vi "MOSES Background 4.vi"(5 "Array Input":refnum<vi>) -> (0 "PSU":dbl[](graph), 1 "Values to Output":T1, 2 "Power Supply Filter Input":dbl[](graph), 3 "ROE":dbl[](graph))   [LabVIEW 2013]
uses:
  Instance          20 26Saved   MOSES Background 4 .vi
  Instance          18 26Saved   MOSES Background 4 .vi
  Instance           7 26Saved   MOSES Background 4 .vi
  Instance          15 26Saved   MOSES Background 4 .vi
  Instance          22 26Saved   MOSES Background 4 .vi
  Instance          13 26Saved   MOSES Background 4 .vi
  Instance          11 26Saved   MOSES Background 4 .vi
  Instance           9 26Saved   MOSES Background 4 .vi
  Instance           5 26Saved   MOSES Background 4 .vi
  Instance           3 26Saved   MOSES Background 4 .vi
  Instance          26 26Saved   MOSES Background 4 .vi
  Instance          25 26Saved   MOSES Background 4 .vi
  Instance          30 26Saved   MOSES Background 4 .vi
  Instance          28 26Saved   MOSES Background 4 .vi
  <vilib>/express/express arith-compare/Formula/XNode/ExpressFormulaBlockNode.xnode
panel:
  out "Boolean 17":bool
  out "Boolean 16":bool
  out "Boolean 15":bool
  out "Boolean 14":bool
  out "Boolean 13":bool
  out "Boolean 41":bool
  out "Boolean 40":bool
  out "Boolean 39":bool
  out "Boolean 38":bool
  out "Boolean 37":bool
  out "Boolean 36":bool
  out "Boolean 35":bool
  out "Boolean 34":bool
  out "Boolean 33":bool
  out "Boolean 32":bool
  out "Boolean 12":bool
  out "Boolean 11":bool
  out "Boolean 10":bool
  out "Boolean 84":bool
  out "Boolean 83":bool
  out "T_PSU, PSU Temp.":dbl
  out "Boolean 82":bool
  out "Boolean 81":bool
  out "T_ROE, ROE Temp.":dbl
  in  "stop 4":bool
  out "ROE_PSI, ROE power supply input current":dbl
  out "ROE_PSV, ROE power supply input voltage":dbl
  out "I_pf5, Premod filter 5V input current":dbl
  out "HAFI, H-alpha filter current":dbl
  out "S28I, Shutter 28V power current":dbl
  out "Ipf12+, Premod filter positive 12V input current":dbl
  out "If_in":dbl[](graph)
  out "Boolean 31":bool
  out "Boolean 30":bool
  out "Boolean 29":bool
  out "If_in, Power supply filter input current":dbl
  out "Boolean 23":bool
  out "Boolean 22":bool
  out "Boolean 9":bool
  out "Boolean 8":bool
  out "Boolean 7":bool
  out "HACV, H-alpha camera voltage":dbl
  out "HAFV, H-alpha filter voltage":dbl
  out "Boolean 21":bool
  out "Boolean 20":bool
  out "Boolean 19":bool
  out "Boolean 18":bool
  out "S28V, Shutter 28V power voltage":dbl
  out "T5V, Thermal 5V power voltage":dbl
  out "V5s, MGA2805S output voltage":dbl
  out "Vina_0y":dbl
  out "Vina_-y":dbl
  out "Vina_+y, INA330 Output":dbl
  out "Vex_0y":dbl
  out "Vex_-y":dbl
  out "Vex_+y":dbl
  out "Va_0y":dbl
  out "Va_-y":dbl
  out "Waveform Chart 2":dbl[](graph)
  out "Va_+y, Thermistor Voltage":dbl
  # "A"
  # "A"
  # "V"
  # "mA"
  # "C"
  # "C"
  # "V"
  # "V"
  # "V"
  # "V"
  # "V"
  # "A"
  # "mA"
  # "mA"
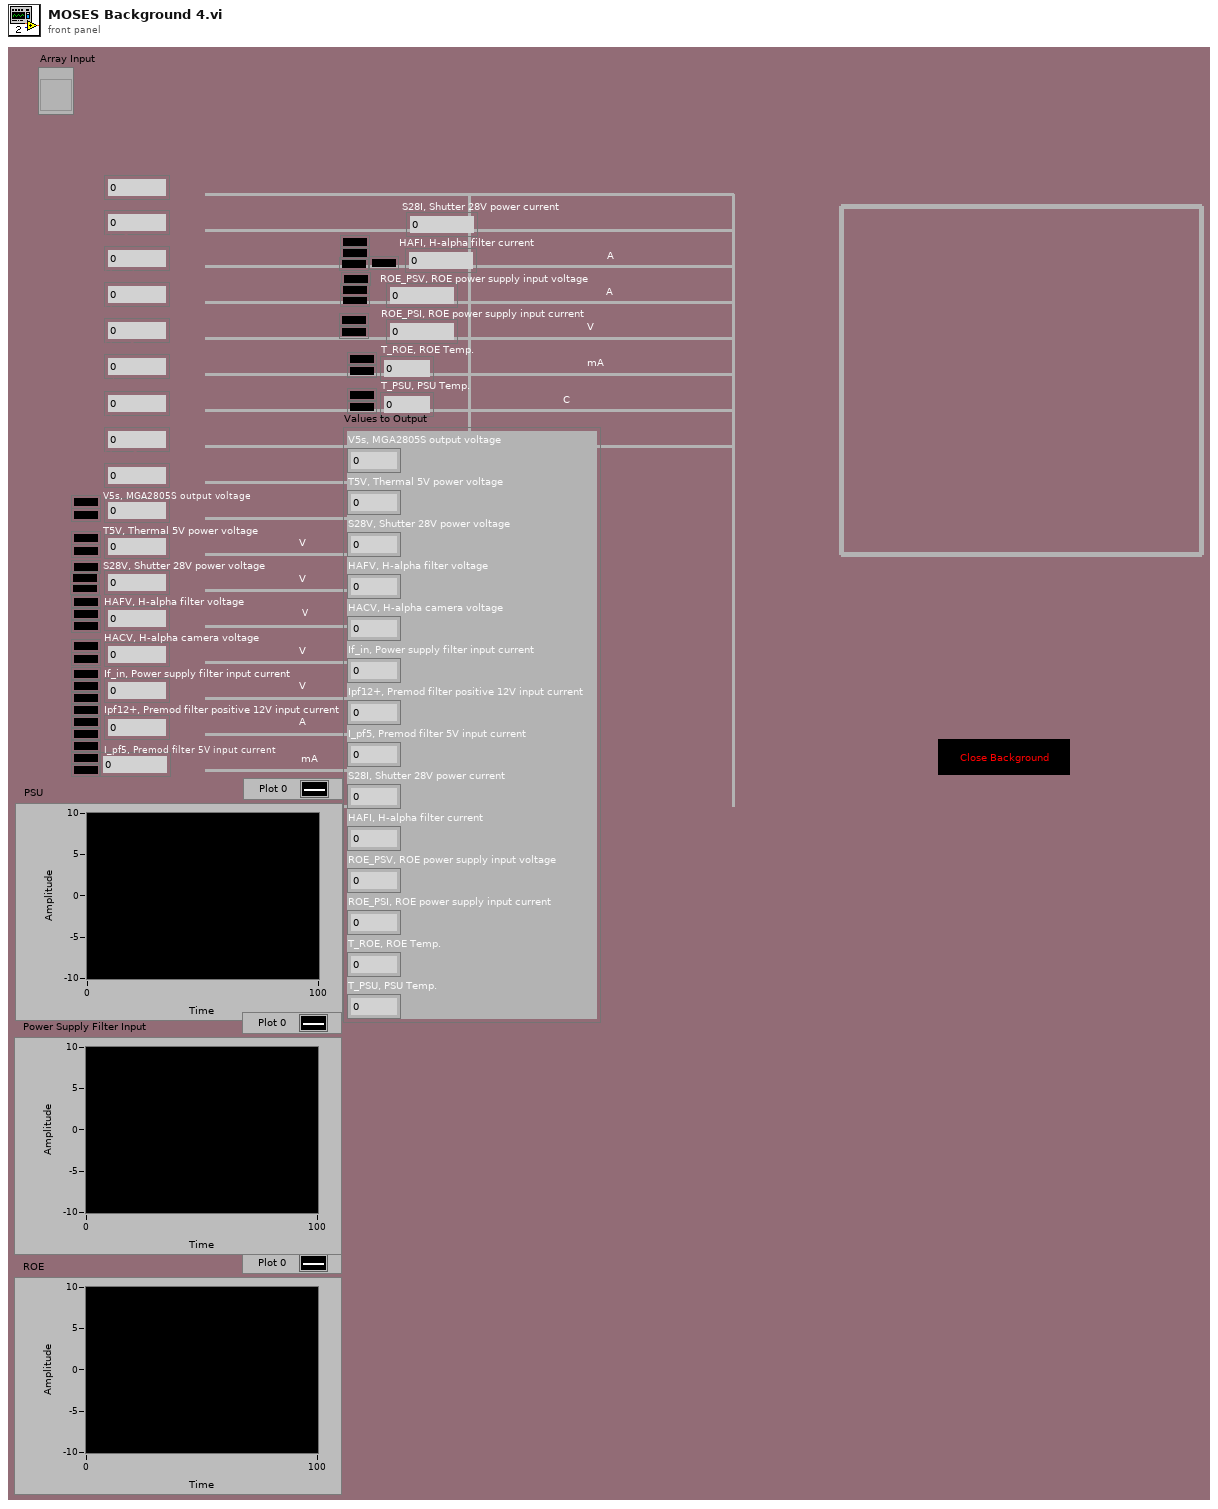
[diagram p1: front panel]
types:
  T1 = cluster{"V5s, MGA2805S output voltage":dbl, "T5V, Thermal 5V power voltage":dbl, "S28V, Shutter 28V power voltage":dbl, "HAFV, H-alpha filter voltage":dbl, "HACV, H-alpha camera voltage":dbl, "If_in, Power supply filter input current":dbl, "Ipf12+, Premod filter positive 12V input current":dbl, "I_pf5, Premod filter 5V input current":dbl, "S28I, Shutter 28V power current":dbl, "HAFI, H-alpha filter current":dbl, "ROE_PSV, ROE power supply input voltage":dbl, "ROE_PSI, ROE power supply input current":dbl, "T_ROE, ROE Temp.":dbl, "T_PSU, PSU Temp.":dbl}
  T2 = cluster{"Value[0]":dbl, "Value[1]":dbl, "Value[2]":dbl, "Value[3]":dbl, "Value[4]":dbl, "Value[5]":dbl, "Value[6]":dbl, "Value[7]":dbl, "Value[8]":dbl, "Value[9]":dbl, "Value[10]":dbl, "Value[11]":dbl, "Value[12]":dbl, "Value[13]":dbl, "Value[14]":dbl, "Value[15]":dbl, "Value[16]":dbl, "Value[17]":dbl, "Value[18]":dbl, "Value[19]":dbl, "Value[20]":dbl, "Value[21]":dbl, "Value[22]":dbl, "Value[23]":dbl, "Value[24]":dbl, "Value[25]":dbl, "Value[26]":dbl, "Value[27]":dbl, "Value[28]":dbl, "Value[29]":dbl, "Value[30]":dbl, "Value[31]":dbl, "Value[32]":dbl, "Value[33]":dbl, "Value[34]":dbl, "Value[35]":dbl, "Value[36]":dbl, "Value[37]":dbl, "Value[38]":dbl, "Value[39]":dbl, "Value[40]":dbl, "Value[41]":dbl, "Value[42]":dbl, "Value[43]":dbl, "Value[44]":dbl, "Value[45]":dbl, "Value[46]":dbl, "Value[47]":dbl, "Value[48]":dbl, "Value[49]":dbl, "Value[50]":dbl, "Value[51]":dbl, "Value[52]":dbl, "Value[53]":dbl, "Value[54]":dbl, "Value[55]":dbl, "Value[56]":dbl, "Value[57]":dbl, "Value[58]":dbl, "Value[59]":dbl, "Value[60]":dbl, "Value[61]":dbl, "Value[62]":dbl, "Value[63]":dbl, "Value[64]":dbl, "Value[65]":dbl, "Value[66]":dbl, "Value[67]":dbl, "Value[68]":dbl, "Value[69]":dbl}
  T3 = cluster{"[0]":dbl, "[1]":dbl, "[2]":dbl, "[3]":dbl, "[4]":dbl, "[5]":dbl, "[6]":dbl, "[7]":dbl, "[8]":dbl, "[9]":dbl, "[10]":dbl, "[11]":dbl, "[12]":dbl, "[13]":dbl}
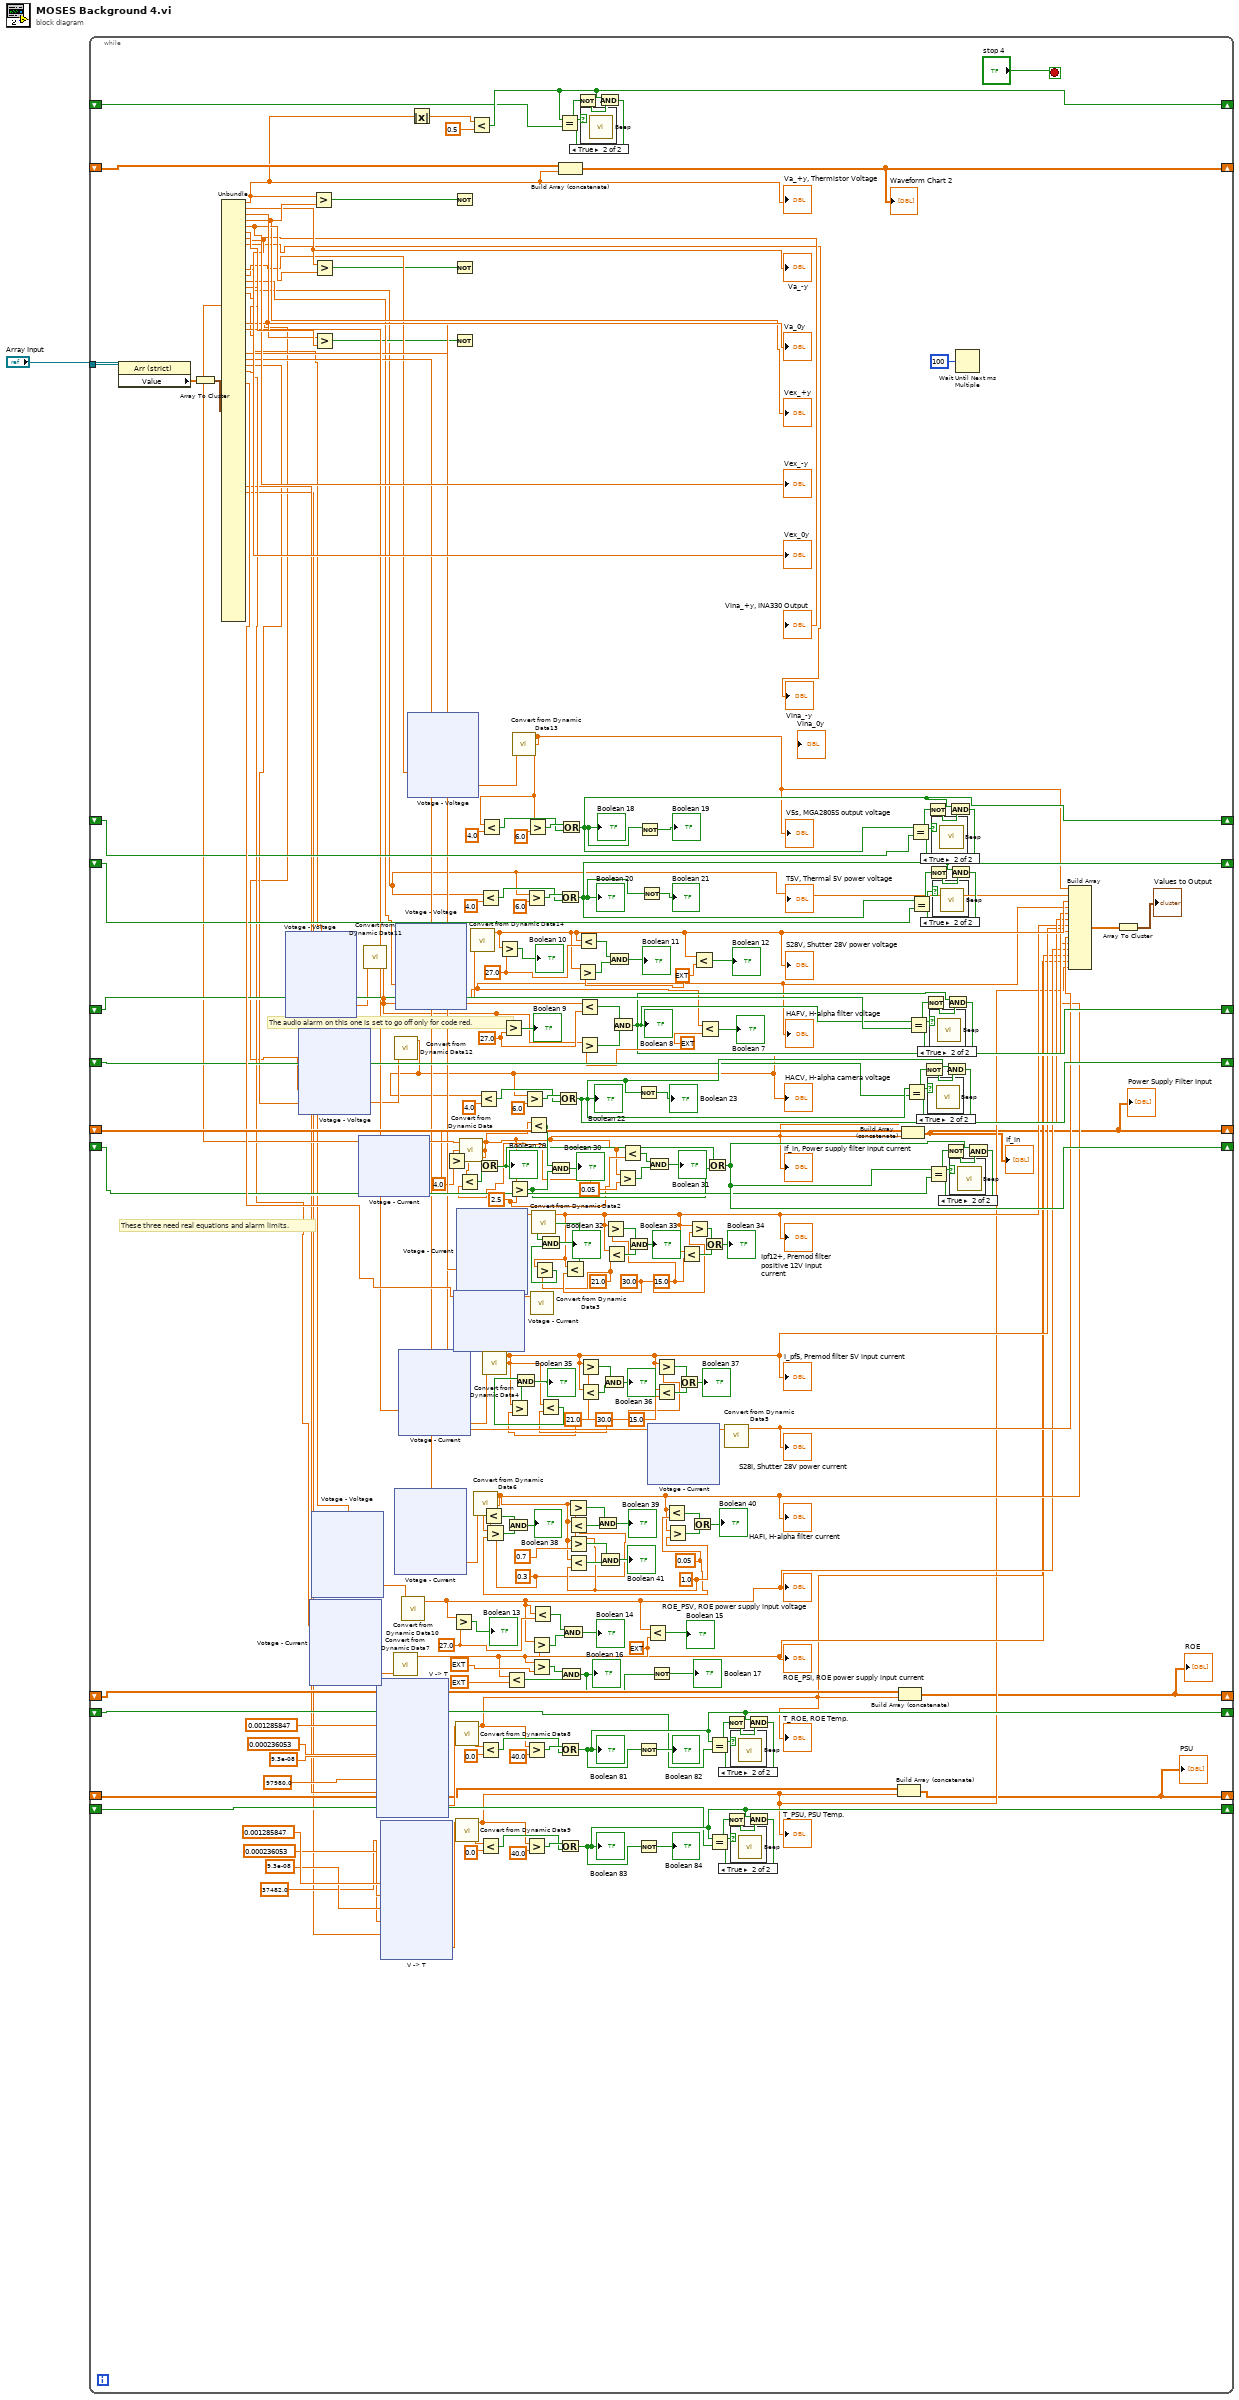
[diagram p0: block diagram]
diagram:
  n1 = while {
    tunnel: "Array Input" -> [w222]
    shift-right: [w218] -> _
    shift-left: _ -> [w219]
    shift-right: [w4] -> _
    shift-left: _ -> [w195]
    shift-right: [w177] -> _
    shift-left: _ -> [w176]
    shift-right: [w160] -> _
    shift-left: _ -> [w159]
    shift-right: [w95] -> _
    shift-left: _ -> [w158]
    shift-right: [w157] -> _
    shift-left: _ -> [w156]
    shift-right: [w155] -> _
    shift-left: _ -> [w154]
    shift-right: [w153] -> _
    shift-left: _ -> [w152]
    shift-right: [w132] -> _
    shift-left: _ -> [w131]
    shift-right: [w130] -> _
    shift-left: _ -> [w129]
    shift-right: [w3] -> _
    shift-left: _ -> [w128]
    shift-right: [w2] -> _
    shift-left: _ -> [w127]
    stop <- "stop 4" stop-if-true
    w41 = 27.0 ("y")
    w36 = ext 20.0 ("y")
    w44 = 0.05 ("y")
    w43 = 0.3 ("y")
    w45 = 1.0 ("y")
    w61 = 15.0 ("y")
    w60 = 30.0 ("y")
    w59 = 21.0 ("y")
    w72 = 15.0 ("y")
    w71 = 30.0 ("y")
    w21 = 21.0 ("y")
    w93 = 27.0 ("y")
    w89 = ext 20.0 ("y")
    w26 = 0.05 ("y")
    w84 = 4.0 ("y")
    w22 = 2.5 ("y")
    w98 = ext 20.0 ("y")
    w202 = 27.0 ("y")
    # "These three need real equations and alarm limits."
    # "The audio alarm on this one is set to go off only for code red."
    n2 = property class="Arr (strict)"(reference=w222) -> ("Value"=w221:dbl[])  [unwired: 1 in, 2 out]
    n3 = Array To Cluster(array=w221) -> (cluster=w220:T2)
    n4 = Unbundle(w220) -> ("Value[0]"=w183:dbl, "Value[1]"=w184:dbl, "Value[2]"=w216:dbl, "Value[3]"=w185:dbl, "Value[4]"=w215:dbl, "Value[5]"=w217:dbl, "Value[6]"=→"Vex_0y" →"Vina_+y, INA330 Output":dbl, "Value[7]"=→"Vina_-y":dbl, "Value[11]"=w101:dbl, "Value[12]"=w19:dbl, "Value[13]"=w99:dbl, "Value[14]"=w103:dbl, "Value[15]"=w105:dbl, "Value[17]"=w124:dbl, "Value[20]"=w123:dbl, "Value[21]"=w122:dbl, "Value[25]"=w121:dbl, "Value[26]"=w120:dbl, "Value[27]"=w107:dbl, "Value[28]"=w119:dbl, "Value[30]"=w192:dbl, "Value[47]"=w110:dbl, "Value[48]"=w109:dbl)  [unwired: 47 out]
    "Va_+y, Thermistor Voltage" <- w183
    "Va_-y" <- w184
    "Va_0y" <- w216
    "Vex_+y" <- w185
    "Vex_-y" <- w215
    "T5V, Thermal 5V power voltage" <- w19
    n5 = xnode "Votage - Voltage"("X1"=w103) -> ("Result"=w104:dbl)  [unwired: 1 in, 1 out]
    n6 = xnode "Votage - Voltage"("X1"=w105) -> ("Result"=w106:dbl)  [unwired: 1 in, 1 out]
    n7 = xnode "Votage - Current"("X1"=w119) -> ("Result"=w188:dbl)  [unwired: 1 in, 1 out]
    n8 = Greater?(x=w183, y=w185) -> (0:w187:bool)
    n9 = xnode "Votage - Voltage"("X1"=w107) -> ("Result"=w108:dbl)  [unwired: 1 in, 1 out]
    n10 = Greater?(x=w184, y=w215) -> (0:w83:bool)
    n11 = Greater?(x=w216, y=w217) -> (0:w82:bool)
    n12 = xnode "Votage - Current"("X1"=w124) -> ("Result"=w196:dbl)  [unwired: 1 in, 1 out]
    n13 = call "Convert from Dynamic Data11"("Dynamic Data Type"=w104) -> ("Scalar"=w17:dbl)  [unwired: 3 in]
    "HAFV, H-alpha filter voltage" <- w17
    n14 = xnode "V -> T"("a"=0.001285847 ("double precision float"), "b"=0.000236053 ("double precision float"), "c"=9.3e-08 ("double precision float"), "R"=97980.0 ("double precision float"), "v0"=w110) -> ("Result"=w145:dbl)  [unwired: 1 in, 1 out]
    n15 = xnode "V -> T"("a"=0.001285847 ("double precision float"), "b"=0.000236053 ("double precision float"), "c"=9.3e-08 ("double precision float"), "R"=37482.0 ("double precision float"), "v0"=w109) -> ("Result"=w136:dbl)  [unwired: 1 in, 1 out]
    n16 = call "Convert from Dynamic Data7"("Dynamic Data Type"=w188) -> ("Scalar"=w9:dbl)  [unwired: 3 in]
    "ROE_PSI, ROE power supply input current" <- w9
    n17 = call "Convert from Dynamic Data12"("Dynamic Data Type"=w106) -> ("Scalar"=w16:dbl)  [unwired: 3 in]
    "HACV, H-alpha camera voltage" <- w16
    n18 = xnode "Votage - Current"("X1"=w120) -> ("Result"=w189:dbl)  [unwired: 1 in, 1 out]
    n19 = xnode "Votage - Voltage"("X1"=w99) -> ("Result"=w100:dbl)  [unwired: 1 in, 1 out]
    n20 = xnode "Votage - Current"("X1"=w122) -> ("Result"=w191:dbl)  [unwired: 1 in, 1 out]
    n21 = call "Convert from Dynamic Data10"("Dynamic Data Type"=w108) -> ("Scalar"=w10:dbl)  [unwired: 3 in]
    "ROE_PSV, ROE power supply input voltage" <- w10
    n22 = xnode "Votage - Voltage"("X1"=w101) -> ("Result"=w102:dbl)  [unwired: 1 in, 1 out]
    n23 = Absolute Value(x=w183) -> (abs(x)=w181:dbl)
    n24 = Greater?(x=w10, y=w41) -> (0:→"Boolean 13":bool)
    n25 = Not(x=w187) -> ()  [unwired: 1 out]
    n26 = Not(x=w83) -> ()  [unwired: 1 out]
    n27 = Not(x=w82) -> ()  [unwired: 1 out]
    n28 = xnode "Votage - Current"("X1"=w192) -> ("Result"=w193:dbl)  [unwired: 1 in, 1 out]
    n29 = call "Convert from Dynamic Data8"("Dynamic Data Type"=w145) -> ("Scalar"=w8:dbl)  [unwired: 3 in]
    "T_ROE, ROE Temp." <- w8
    n30 = call "Convert from Dynamic Data9"("Dynamic Data Type"=w136) -> ("Scalar"=w7:dbl)  [unwired: 3 in]
    "T_PSU, PSU Temp." <- w7
    n31 = xnode "Votage - Current"("X1"=w123) -> ("Result"=w194:dbl)  [unwired: 1 in, 1 out]
    n32 = call "Convert from Dynamic Data"("Dynamic Data Type"=w196) -> ("Scalar"=w15:dbl)  [unwired: 3 in]
    "If_in, Power supply filter input current" <- w15
    n33 = Greater?(x=w15, y=w84) -> (0:w27:bool)
    n34 = Less?(x=w15, y=w26) -> (x < y?=w29:bool)
    n35 = Less?(x=w181, y=0.5) -> (x < y?=w177:bool)
    n36 = call "Convert from Dynamic Data14"("Dynamic Data Type"=w100) -> ("Scalar"=w18:dbl)  [unwired: 3 in]
    "S28V, Shutter 28V power voltage" <- w18
    n37 = call "Convert from Dynamic Data6"("Dynamic Data Type"=w189) -> ("Scalar"=w11:dbl)  [unwired: 3 in]
    "HAFI, H-alpha filter current" <- w11
    n38 = Less?(x=w16, y=4.0) -> (x < y?=w198:bool)
    n39 = Or(x=w27, y=w29) -> (x .or. y?=w28:bool)
    "Boolean 29" <- w28
    n40 = Less?(x=w19, y=4.0) -> (x < y?=w206:bool)
    n41 = Less?(x=w8, y=0.0) -> (x < y?=w147:bool)
    n42 = Less?(x=w7, y=0.0) -> (x < y?=w138:bool)
    n43 = Less?(x=w11, y=w43) -> (x < y?=w57:bool)
    n44 = call "Convert from Dynamic Data4"("Dynamic Data Type"=w191) -> ("Scalar"=w13:dbl)  [unwired: 3 in]
    "I_pf5, Premod filter 5V input current" <- w13
    n45 = Greater?(x=w11, y=w44) -> (0:w58:bool)
    n46 = Greater?(x=w18, y=w93) -> (0:→"Boolean 10":bool)
    n47 = Greater?(x=w17, y=w202) -> (0:→"Boolean 9":bool)
    n48 = Less?(x=w9, y=ext 390.0) -> (x < y?=w33:bool)
    n49 = And(x=w57, y=w58) -> (x .and. y?=→"Boolean 38":bool)
    n50 = Greater?(x=w15, y=w22) -> (0:w87:bool)
    n51 = Greater?(x=w13, y=w59) -> (0:w70:bool)
    n52 = call "Convert from Dynamic Data13"("Dynamic Data Type"=w102) -> ("Scalar"=w20:dbl)  [unwired: 3 in]
    "V5s, MGA2805S output voltage" <- w20
    n53 = Less?(x=w20, y=4.0) -> (x < y?=w211:bool)
    n54 = Greater?(x=w16, y=6.0) -> (0:w199:bool)
    n55 = Greater?(x=w19, y=6.0) -> (0:w207:bool)
    n56 = Greater?(x=w8, y=40.0) -> (0:w148:bool)
    n57 = Greater?(x=w7, y=40.0) -> (0:w139:bool)
    n58 = Greater?(x=w20, y=6.0) -> (0:w212:bool)
    n59 = Less?(x=w15, y=w84) -> (x < y?=w85:bool)
    n60 = Greater?(x=w9, y=ext 250.0) -> (0:w32:bool)
    n61 = call "Convert from Dynamic Data3"("Dynamic Data Type"=w193) -> ()  [unwired: 3 in, 1 out]
    n62 = Greater?(x=w10, y=w36) -> (0:w40:bool)
    n63 = Less?(x=w10, y=w41) -> (x < y?=w39:bool)
    n64 = call "Convert from Dynamic Data2"("Dynamic Data Type"=w194) -> ("Scalar"=w14:dbl)  [unwired: 3 in]
    "Ipf12+, Premod filter positive 12V input current" <- w14
    n65 = Greater?(x=w14, y=w21) -> (0:w81:bool)
    n66 = Less?(x=w13, y=w60) -> (x < y?=w69:bool)
    n67 = And(x=w69, y=w70) -> (x .and. y?=→"Boolean 35":bool)
    n68 = And(x=w85, y=w87) -> (x .and. y?=→"Boolean 30":bool)
    n69 = Or(x=w199, y=w198) -> (x .or. y?=w160:bool)
    "Boolean 22" <- w160
    n70 = Equal?(x=w177, y=w176) -> (x = y?=w178:bool)
    n71 = Build Array (concatenate)(w219, w183) -> (w218:dbl[])
    "Waveform Chart 2" <- w218
    n72 = Or(x=w207, y=w206) -> (x .or. y?=w157:bool)
    "Boolean 20" <- w157
    n73 = Or(x=w148, y=w147) -> (x .or. y?=w132:bool)
    "Boolean 81" <- w132
    n74 = Or(x=w139, y=w138) -> (x .or. y?=w130:bool)
    "Boolean 83" <- w130
    n75 = Or(x=w212, y=w211) -> (x .or. y?=w155:bool)
    "Boolean 18" <- w155
    n76 = And(x=w32, y=w33) -> (x .and. y?=w31:bool)
    "Boolean 16" <- w31
    n77 = And(x=w39, y=w40) -> (x .and. y?=→"Boolean 14":bool)
    n78 = Less?(x=w14, y=w71) -> (x < y?=w80:bool)
    n79 = And(x=w80, y=w81) -> (x .and. y?=→"Boolean 32":bool)
    n80 = Greater?(x=w11, y=w43) -> (0:w55:bool)
    n81 = Less?(x=w11, y=w45) -> (x < y?=w54:bool)
    n82 = Greater?(x=w11, y=0.7) -> (0:w51:bool)
    n83 = Less?(x=w11, y=w45) -> (x < y?=w52:bool)
    n84 = Not(x=w178) -> (.not. x?=w179:bool)
    n85 = Greater?(x=w18, y=w89) -> (0:w92:bool)
    n86 = Less?(x=w18, y=w93) -> (x < y?=w91:bool)
    n87 = Less?(x=w17, y=w202) -> (x < y?=w97:bool)
    n88 = Greater?(x=w17, y=w98) -> (0:w96:bool)
    n89 = Greater?(x=w13, y=w61) -> (0:w66:bool)
    n90 = Less?(x=w13, y=w59) -> (x < y?=w67:bool)
    n91 = And(x=w55, y=w54) -> (x .and. y?=→"Boolean 39":bool)
    n92 = And(x=w177, y=w179) -> (x .and. y?=w180:bool)
    n93 = case shown="True" w180 {
      frame False {
      }
      frame True {
        n94 = call <vilib>:"Beep.vi"() -> ()  [unwired: 12 in]
      }
    }
    n95 = And(x=w51, y=w52) -> (x .and. y?=→"Boolean 41":bool)
    n96 = And(x=w66, y=w67) -> (x .and. y?=→"Boolean 36":bool)
    n97 = Greater?(x=w14, y=w72) -> (0:w77:bool)
    n98 = Less?(x=w14, y=w21) -> (x < y?=w76:bool)
    n99 = And(x=w91, y=w92) -> (x .and. y?=→"Boolean 11":bool)
    n100 = And(x=w97, y=w96) -> (x .and. y?=w95:bool)
    "Boolean 8" <- w95
    n101 = Greater?(x=w15, y=w26) -> (0:w25:bool)
    n102 = Less?(x=w15, y=w22) -> (x < y?=w23:bool)
    n103 = And(x=w77, y=w76) -> (x .and. y?=→"Boolean 33":bool)
    n104 = Not(x=w160) -> (.not. x?=→"Boolean 23":bool)
    n105 = Not(x=w132) -> (.not. x?=→"Boolean 82":bool)
    n106 = Not(x=w130) -> (.not. x?=→"Boolean 84":bool)
    n107 = Not(x=w155) -> (.not. x?=→"Boolean 19":bool)
    n108 = Not(x=w157) -> (.not. x?=→"Boolean 21":bool)
    n109 = Less?(x=w10, y=w36) -> (x < y?=→"Boolean 15":bool)
    n110 = And(x=w23, y=w25) -> (x .and. y?=→"Boolean 31":bool)
    n111 = xnode "Votage - Current"("X1"=w121) -> ("Result"=w190:dbl)  [unwired: 1 in, 1 out]
    n112 = Not(x=w31) -> (.not. x?=→"Boolean 17":bool)
    n113 = Greater?(x=w13, y=w60) -> (0:w63:bool)
    n114 = Less?(x=w13, y=w61) -> (x < y?=w64:bool)
    n115 = Less?(x=w11, y=w44) -> (x < y?=w48:bool)
    n116 = Greater?(x=w11, y=w45) -> (0:w49:bool)
    n117 = Or(x=w63, y=w64) -> (x .or. y?=→"Boolean 37":bool)
    n118 = Less?(x=w14, y=w72) -> (x < y?=w74:bool)
    n119 = Greater?(x=w14, y=w71) -> (0:w73:bool)
    n120 = Or(x=w48, y=w49) -> (x .or. y?=→"Boolean 40":bool)
    n121 = Less?(x=w18, y=w89) -> (x < y?=→"Boolean 12":bool)
    n122 = Less?(x=w17, y=w98) -> (x < y?=→"Boolean 7":bool)
    n123 = Or(x=w73, y=w74) -> (x .or. y?=→"Boolean 34":bool)
    n124 = Or(x=w28, y=w87) -> (x .or. y?=w153:bool)
    n125 = Equal?(x=w132, y=w131) -> (x = y?=w142:bool)
    n126 = Equal?(x=w130, y=w129) -> (x = y?=w133:bool)
    n127 = call "Convert from Dynamic Data5"("Dynamic Data Type"=w190) -> ("Scalar"=w12:dbl)  [unwired: 3 in]
    "S28I, Shutter 28V power current" <- w12
    n128 = Not(x=w142) -> (.not. x?=w143:bool)
    n129 = Not(x=w133) -> (.not. x?=w134:bool)
    n130 = And(x=w132, y=w143) -> (x .and. y?=w144:bool)
    n131 = case shown="True" w144 {
      frame False {
      }
      frame True {
        n132 = call <vilib>:"Beep.vi"() -> ()  [unwired: 12 in]
      }
    }
    n133 = And(x=w130, y=w134) -> (x .and. y?=w135:bool)
    n134 = case shown="True" w135 {
      frame False {
      }
      frame True {
        n135 = call <vilib>:"Beep.vi"() -> ()  [unwired: 12 in]
      }
    }
    n136 = Build Array (concatenate)(w127, w7) -> (w2:dbl[])
    "PSU" <- w2
    n137 = Build Array (concatenate)(w128, w8) -> (w3:dbl[])
    "ROE" <- w3
    n138 = Build Array (concatenate)(w195, w15) -> (w4:dbl[])
    "If_in" <- w4
    "Power Supply Filter Input" <- w4
    n139 = Equal?(x=w160, y=w159) -> (x = y?=w164:bool)
    n140 = Equal?(x=w95, y=w158) -> (x = y?=w167:bool)
    n141 = Equal?(x=w155, y=w154) -> (x = y?=w173:bool)
    n142 = Equal?(x=w157, y=w156) -> (x = y?=w170:bool)
    n143 = Not(x=w164) -> (.not. x?=w165:bool)
    n144 = Not(x=w167) -> (.not. x?=w168:bool)
    n145 = Not(x=w173) -> (.not. x?=w174:bool)
    n146 = Not(x=w170) -> (.not. x?=w171:bool)
    n147 = Equal?(x=w153, y=w152) -> (x = y?=w161:bool)
    n148 = Not(x=w161) -> (.not. x?=w162:bool)
    n149 = And(x=w160, y=w165) -> (x .and. y?=w166:bool)
    n150 = case shown="True" w166 {
      frame False {
      }
      frame True {
        n151 = call <vilib>:"Beep.vi"() -> ()  [unwired: 12 in]
      }
    }
    n152 = And(x=w95, y=w168) -> (x .and. y?=w169:bool)
    n153 = case shown="True" w169 {
      frame False {
      }
      frame True {
        n154 = call <vilib>:"Beep.vi"() -> ()  [unwired: 12 in]
      }
    }
    n155 = And(x=w155, y=w174) -> (x .and. y?=w175:bool)
    n156 = case shown="True" w175 {
      frame False {
      }
      frame True {
        n157 = call <vilib>:"Beep.vi"() -> ()  [unwired: 12 in]
      }
    }
    n158 = And(x=w157, y=w171) -> (x .and. y?=w172:bool)
    n159 = case shown="True" w172 {
      frame False {
      }
      frame True {
        n160 = call <vilib>:"Beep.vi"() -> ()  [unwired: 12 in]
      }
    }
    n161 = Wait Until Next ms Multiple(millisecond multiple=u32 100) -> ()  [unwired: 1 out]
    n162 = And(x=w153, y=w162) -> (x .and. y?=w163:bool)
    n163 = case shown="True" w163 {
      frame False {
      }
      frame True {
        n164 = call <vilib>:"Beep.vi"() -> ()  [unwired: 12 in]
      }
    }
    n165 = Build Array(w20, w19, w18, w17, w16, w15, w14, w13, w12, w11, w10, w9, w8, w7) -> (w6:dbl[])
    n166 = Array To Cluster(array=w6) -> (cluster=→"Values to Output":T3)
  }
